vi "Get Characterization Frequencies.vi"(0 "VISA resource name":refnum<visa-resource-name>, 11 "error in (no error)":errorcluster) -> (4 "VISA resource name out":refnum<visa-resource-name>, 8 "S-Par Characterization Frequencies":dbl[](array[numeric]), 15 "error out":errorcluster)   [LabVIEW 2023, in "ACM Visa Driver.lvlib"]
uses:
  ACM Visa Driver.lvlib
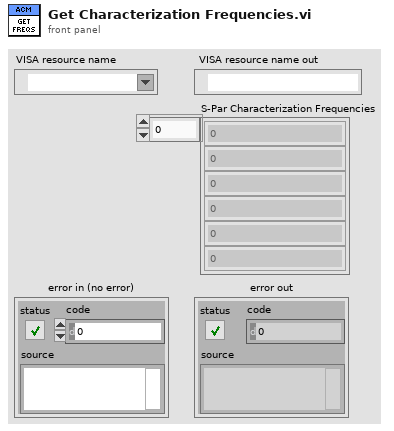
[diagram p1: front panel]
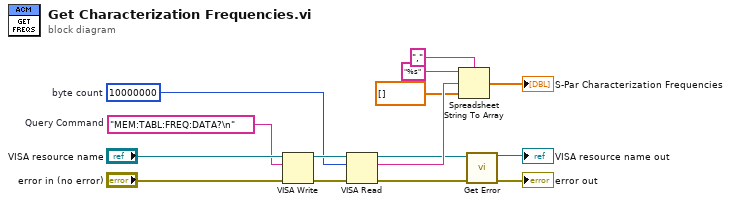
[diagram p0: block diagram]
diagram:
  w4 = u32 10000000  # byte count
  w6 = "MEM:TABL:FREQ:DATA?\n"  # Query Command
  n1 = VISA Write(VISA resource name="VISA resource name", write buffer=w6, error in (no error)="error in (no error)") -> (VISA resource name out=w12:refnum<visa-resource-name>, error out=w14:errorcluster)  [unwired: 1 out]
  n2 = VISA Read(VISA resource name=w12, byte count=w4, error in (no error)=w14) -> (VISA resource name out=w2:refnum<visa-resource-name>, read buffer=w10:string, error out=w13:errorcluster)  [unwired: 1 out]
  n3 = Spreadsheet String To Array(delimiter (Tab)=",", format string="%s", spreadsheet string=w10, array type (2D Dbl)=dbl[] []) -> (array=→"S-Par Characterization Frequencies":dbl[])
  n4 = call "Get Error.vi"("VISA resource name"=w2, "error in (no error)"=w13) -> ("VISA resource name out"=→"VISA resource name out":refnum<visa-resource-name>, "error out"=→"error out":errorcluster)  [unwired: 12 in]
